vi "fpga_MagnitudePhase (M Class).vi"(0 "re":fxp<+/-,32,6> format="%.29g", 1 "reset":bool, 2 "filter delay constant":T1, 5 "im":fxp<+/-,32,6> format="%.29g", 7 "Ch":fxp<+,5,5>=6.0, 9 "input valid":bool, 12 "ready for output":bool) -> (4 "rms magnitude":fxp<+,32,6> format="%.28g", 6 "phase":fxp<+/-,32,2> format="%.31g", 10 "output valid":bool, 14 "ready for input":bool)   [LabVIEW 2013, in "NI_EP_PMU_FPGA.lvlib"]
uses:
  <vilib>/addons/Electrical Power/PMU/NI_EP_PMU_FPGA.lvlib
  <vilib>/addons/Electrical Power/PMU/FPGA/subVIs/fpga_Reporting Rate Configuration.ctl
  <vilib>/rvi/FXPMathLib/FxpRectToPolar/subVIs/nifxpmath_RectToPolar_SimConfig.ctl
  <vilib>/rvi/Emulation/niFpgaSctlEmulationGetInTimedLoop.vi
  <vilib>/rvi/eio/common/nirviEmuReportErrorAndStop.vi
  <vilib>/rvi/DataTransferAndStorage/Container/Common/niFpgaContainerSetEmuInfo.vi
  <vilib>/rvi/DataTransferAndStorage/Container/Common/niFpgaContainerGetUniqueNameForEmu.vi
  <vilib>/rvi/FXPMathLib/FxpRectToPolar/simVIs/DllFxpRectToPolarTemp_sub.vi
  <vilib>/rvi/Memory/Memory_Emulation/nirvimemoryEmulation.vi
  <vilib>/rvi/Memory/Memory_Emulation/nirvimemoryFastEmulation.vi
  <vilib>/rvi/Memory/Memory_Emulation/nirvimemoryEmulationManagerCache_ReleaseExclusive.vi
  <vilib>/rvi/Memory/Memory_Emulation/niFpgaMemoryEmulationValidateCache.vi
  <vilib>/rvi/Memory/Memory_Emulation/nirvimemoryEmulationManagerCache_MakeExclusive.vi
  <vilib>/rvi/Memory/Memory_Emulation/niFpgaMemoryEmulationCacheClearOnFirstRun.vi
  <vilib>/rvi/Memory/Memory_Emulation/nirvimemoryEmulationManagerCache_InsertValue.vi
  <vilib>/Utility/error.llb/Clear Errors.vi
  <vilib>/rvi/Memory/Memory_Emulation/nirvimemoryEmulationManagerCache_GetValue.vi
  <vilib>/rvi/LocalResourceManager/LocalResourceManager.xnode
  <vilib>/rvi/FXPMathLib/FxpRectToPolar/XNode/nifxpmath_RectToPolar.xnode
  <vilib>/rvi/FXPMathLib/basic elements/FxpDiscreteDelay/XNode/nifxpmath_DiscreteDelay.xnode
  <vilib>/rvi/DataTransferAndStorage/Container/XNode/niFpgaContainer.xnode
  <vilib>/rvi/FXPMathLib/FxpAdd/XNode/nifxpmath_Add.xnode
  <vilib>/addons/Electrical Power/PQ/Resampling/NI_EP_Resample_FPGA.lvlib
  <vilib>/rvi/FXPMathLib/sim/FxpSim.dll
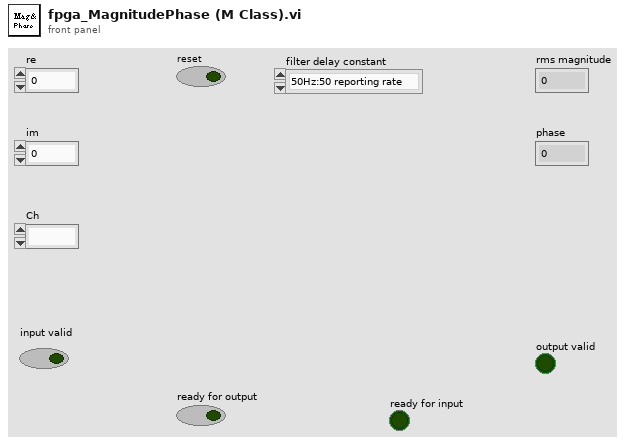
[diagram p1: front panel]
types:
  T1 = typedef "NI_EP_PMU_FPGA.lvlib/fpga_Reporting Rate Configuration.ctl" = enum16{"50Hz:50 reporting rate", "50Hz:25 reporting rate", "50Hz:10 reporting rate", "60Hz:60 reporting rate", "60Hz:30 reporting rate", "60Hz:20 reporting rate", "60Hz:15 reporting rate", "60Hz:12 reporting rate", "60Hz:10 reporting rate"}
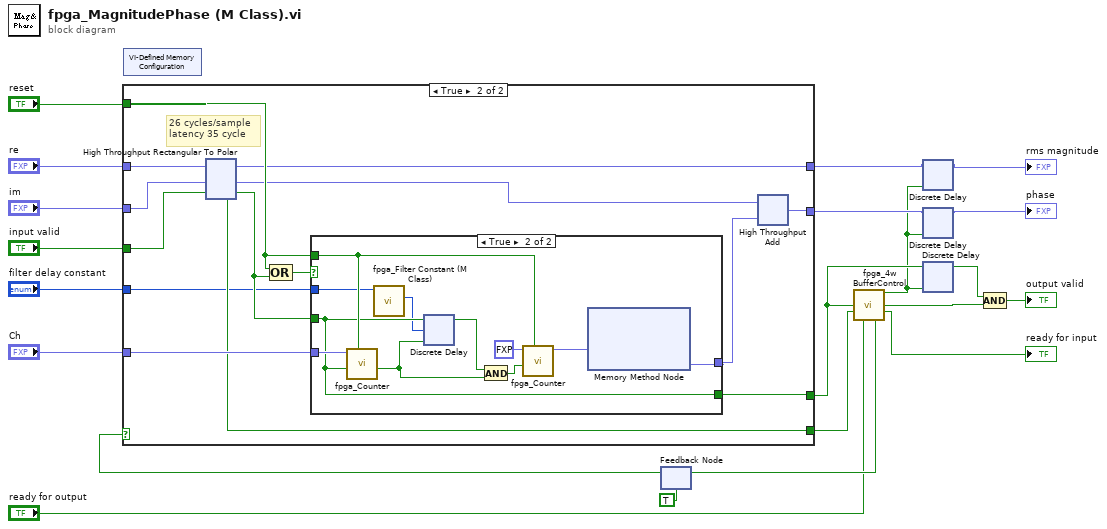
[diagram p0: block diagram]
diagram:
  n1 = xnode "VI-Defined Memory Configuration"() -> ()  [unwired: 1 out]
  n2 = feedback #1(TRUE ("logic enable")) -> (w17:bool)
  n3 = case shown="True" w17 {
    tunnel: "input valid" -> [_ w31]
    tunnel: "reset" -> [_ w30]
    tunnel: "Ch" -> [_ w29]
    tunnel: "re" -> [_ w33]
    tunnel: "im" -> [_ w32]
    tunnel: [_ w26] -> w8
    tunnel: [_ w27] -> w9
    tunnel: [_ w28] -> w6
    tunnel: [_ w23] -> w4
    tunnel: "filter delay constant" -> [_ w22]
    frame False {
    }
    frame True {
      # "26 cycles/sample\nlatency 35 cycle"
      n4 = xnode "High Throughput Rectangular To Polar"("x"=w33, "y"=w32, "input valid"=w31) -> ("magnitude"=w23:fxp<+,32,6>, "phase (pi)"=w24:fxp<+/-,32,2>, "output valid"=w34:bool, "ready for input"=w27:bool)  [unwired: 1 in]
      n5 = Compound Arithmetic op=OR(w30, w34) -> (w35:bool)
      n6 = case shown="True" w35 {
        tunnel: [_ w46] -> w25
        tunnel: [_ w39] -> w26
        tunnel: w29 -> [_ w45]
        tunnel: w34 -> [_ w39]
        tunnel: w30 -> [_ w44]
        tunnel: w22 -> [_ w36]
        frame False {
        }
        frame True {
          n7 = call <vilib>:"fpga_Counter.vi"("reset"=w44, "Input Valid?"=w39, "upper limit"=w45) -> ("Multichannel Valid?"=w40:bool)  [unwired: 7 in, 1 out]
          n8 = call <vilib>:"fpga_Filter Constant (M Class).vi"("filter delay constant"=w36) -> ("LP2 delay"=w37:u8)  [unwired: 6 in, 4 out]
          n9 = xnode ("Discrete Delay")("D"=w39, "n-1[0..23]"=w37, "enable"=w40) -> ("Q"=w38:bool)
          n10 = And(x=w38, y=w40) -> (x .and. y?=w43:bool)
          n11 = call <vilib>:"fpga_Counter.vi"("reset"=w44, "Input Valid?"=w43, "upper limit"=fxp<+,5,5> 24.0 ("#ch")) -> ("count"=w42:fxp<+,5,5>)  [unwired: 7 in, 1 out]
          n12 = xnode ("Memory Method Node")("Address"=w42) -> ("Data"=w46:fxp<+/-,32,2>)  [unwired: 1 in, 1 out]
        }
      }
      n13 = xnode ("High Throughput Add")("x"=w24, "y"=w25) -> ("x+y"=w28:fxp<+/-,32,2>)
    }
  }
  n14 = call <vilib>:"fpga_4w BufferControl.vi"("DR"=w8, "RFI"=w9, "RFO"="ready for output") -> ("buff enable"=w3:bool, "output valid"=w19:bool, "ready for input"=→"ready for input":bool, "logic enable"=w18:bool)  [unwired: 9 in]
  n15 = feedback-in #1(w18) -> ()
  n16 = xnode ("Discrete Delay")("D"=w4, "enable"=w3) -> ("Q"=→"rms magnitude":fxp<+,32,6>)
  n17 = xnode ("Discrete Delay")("D"=w6, "enable"=w3) -> ("Q"=→"phase":fxp<+/-,32,2>)
  n18 = xnode ("Discrete Delay")("D"=w8, "enable"=w3) -> ("Q"=w7:bool)
  n19 = Compound Arithmetic op=AND(w7, w19) -> (→"output valid":bool)
